vi "CreateRandom.vi"(8 "error in (no error)":errorcluster, 9 "Col":i32, 10 "Row":i32, 11 "MCListbox Refnum":refnum<vi>) -> (0 "error out":errorcluster)   [LabVIEW 2011]
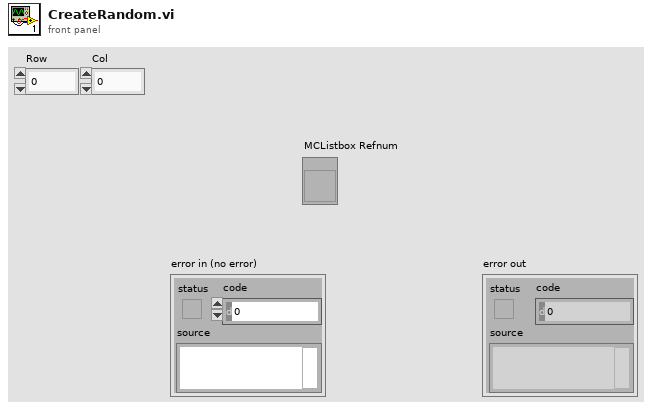
[diagram p1: front panel]
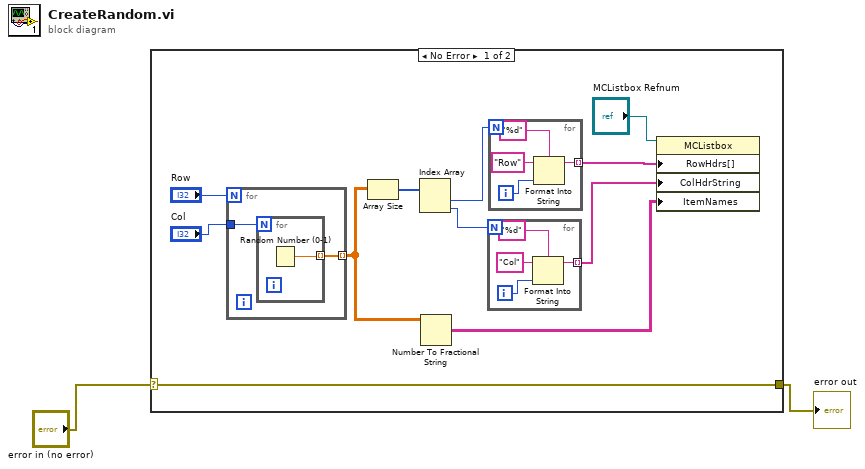
[diagram p0: block diagram]
diagram:
  n1 = case shown="No Error" "error in (no error)" {
    selector: "error in (no error)" -> [w13 w25]
    tunnel: [w13 w25] -> w1
    frame No Error {
      n2 = for {
        N: "Row" -> [_]
        tunnel: "Col" -> [w23]
        tunnel: [w22] -> w10 mode=indexing
        n3 = for {
          N: w23 -> [_]
          tunnel: [w24] -> w22 mode=indexing
          n4 = Random Number (0-1)() -> (number: 0 to 1=w24:dbl)
        }
      }
      n5 = Array Size(array=w10) -> (size(s)=w8:i32[])
      n6 = Index Array(array=w8) -> (element #1=w6:i32, element #2=w4:i32)  [unwired: 2 in]
      n7 = Number To Fractional String(number=w10) -> (F-format string=w3:string[][])  [unwired: 3 in]
      n8 = for {
        N: w4 -> [_]
        tunnel: [w14] -> w5 mode=indexing
        i -> [w17]
        n9 = Format Into String(format string="%d", initial string="Col", w17) -> (resulting string=w14:string)  [unwired: 1 in, 1 out]
      }
      n10 = for {
        N: w6 -> [_]
        tunnel: [w18] -> w7 mode=indexing
        i -> [w21]
        n11 = Format Into String(format string="%d", initial string="Row", w21) -> (resulting string=w18:string)  [unwired: 1 in, 1 out]
      }
      n12 = property class="MCListbox"(reference="MCListbox Refnum", "RowHdrs[]"=w7, "ColHdrString"=w5, "ItemNames"=w3) -> ()  [unwired: 1 in, 2 out]
    }
    frame Error {
    }
  }
  "error out" <- w1
